vi "Sets the IR LO SET resistance value for MANU.vi"(5 "Enable to Query":bool, 7 "Enable to Setup":bool, 8 "error in":errorcluster, 10 "IR LO SET resistance value(M£[)":u16=2 min=1 max=9999, 11 "VISA resource name":refnum<visa-resource-name>) -> (0 "error out":errorcluster, 2 "Return the IR LO SET resistance value":string, 3 "VISA resource name out":refnum<visa-resource-name>)   [LabVIEW 2011, in "GPT-9000.lvlib"]
uses:
  <instrlib>/GPT-9000/GPT-9000.lvlib
panel:
  # "M£["
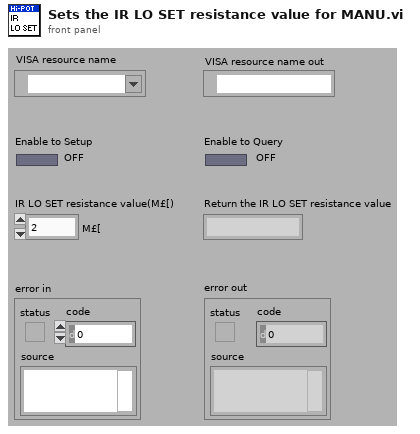
[diagram p1: front panel]
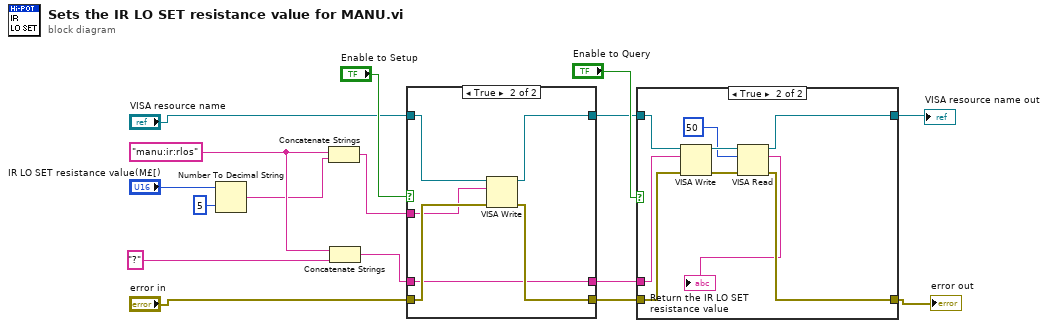
[diagram p0: block diagram]
diagram:
  w15 = "manu:ir:rlos"
  n1 = Number To Decimal String(number="IR LO SET resistance value(M£[)", width (-)=i16 5) -> (decimal integer string=w1:string)
  n2 = Concatenate Strings(w15, w1) -> (w13:string)
  n3 = Concatenate Strings(w15, "?") -> (w12:string)
  n4 = case shown="True" "Enable to Setup" {
    tunnel: w13 -> [_ w20]
    tunnel: w12 -> [w17 w21]
    tunnel: "VISA resource name" -> [w19 w25]
    tunnel: "error in" -> [w18 w24]
    tunnel: [w19 w23] -> w8
    tunnel: [w18 w22] -> w7
    tunnel: [w17 w21] -> w6
    frame False {
    }
    frame True {
      n5 = VISA Write(VISA resource name=w25, write buffer=w20, error in (no error)=w24) -> (VISA resource name out=w23:refnum<visa-resource-name>, error out=w22:errorcluster)  [unwired: 1 out]
    }
  }
  n6 = case shown="True" "Enable to Query" {
    tunnel: w8 -> [w27 w35]
    tunnel: w7 -> [w26 w34]
    tunnel: w6 -> [_ w36]
    tunnel: [w27 w30] -> w5
    tunnel: [w26 w29] -> w4
    frame False {
    }
    frame True {
      n7 = VISA Write(VISA resource name=w35, write buffer=w36, error in (no error)=w34) -> (VISA resource name out=w32:refnum<visa-resource-name>, error out=w33:errorcluster)  [unwired: 1 out]
      n8 = VISA Read(VISA resource name=w32, byte count=u32 50, error in (no error)=w33) -> (VISA resource name out=w30:refnum<visa-resource-name>, read buffer=→"Return the IR LO SET resistance value":string, error out=w29:errorcluster)  [unwired: 1 out]
    }
  }
  "VISA resource name out" <- w5
  "error out" <- w4
